vi "Touch_Text.vi"(8 "Error In":errorcluster, 11 "TextTouch":string) -> (0 "error out":errorcluster, 3 "Image":T1(plugin-control))   [LabVIEW 2025]
uses:
  Controls/TextTouch.ctl
  Controls/Text2Img.ctl
  Controls/TouchXY.ctl
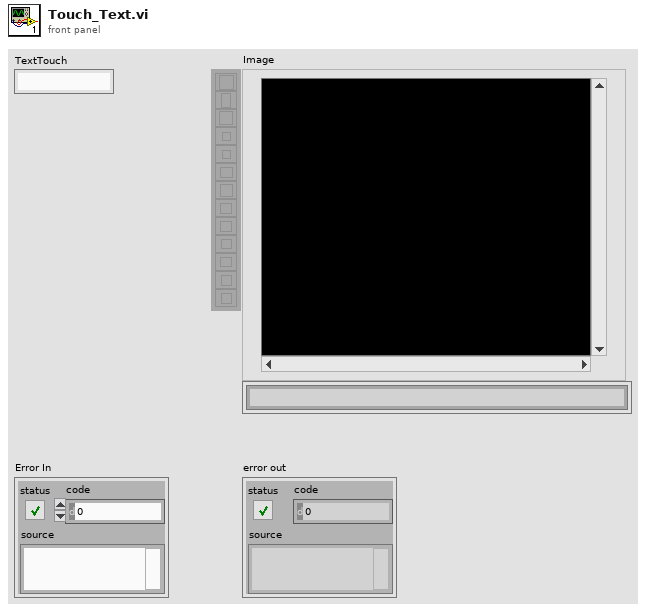
[diagram p1: front panel]
types:
  T1 = typedef "IMAQ Image.ctl" = refnum<image>
  T2 = typedef "TextTouch.ctl" = cluster{"Match%":dbl, "ROI":cluster{"Global Rectangle":i32[], "Contours":cluster{"Contour Type":u32, "ROI Type":u32, "Points":i32[]}[]}, "TextInfo":cluster{"Text":string, "TextColor":cluster{"Text BG":u32, "Text Color":u32}, "Size":u16, "FontDetails":T3}}
  T3 = typedef "Text2Img.ctl" = cluster{"Text.Font":cluster{"Font Name":string, "Size":u16, "Bold":bool, "Italic":bool, "Underline":bool, "Strikeout":bool, "Color":u32}}
  T4 = cluster{"Global Rectangle":i32[], "Contours":cluster{"Contour Type":u32, "ROI Type":u32, "Points":i32[]}[]}
  T5 = cluster{"Text":string, "TextColor":cluster{"Text BG":u32, "Text Color":u32}, "Size":u16, "FontDetails":T3}
  T6 = typedef "TouchXY.ctl" = cluster{"Win Name":string, "TouchCoord":cluster{"x":sgl, "y":sgl}}
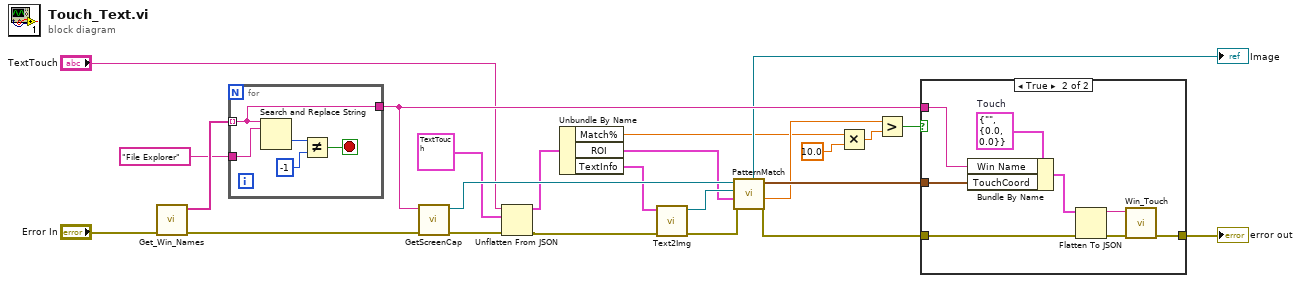
[diagram p0: block diagram]
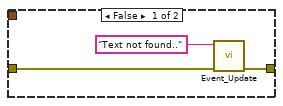
[diagram p2: hidden frame]
diagram:
  n1 = call "Get_Win_Names.vi"("error in"="Error In") -> ("Win_Names"=w23:string[], "error out"=w20:errorcluster)  [unwired: 8 in]
  n2 = for {
    tunnel: w23 -> [w26] mode=indexing
    tunnel: "File Explorer" ("Win Name") -> [w29]
    tunnel: [w26] -> w21
    stop <- w27 stop-if-true
    n3 = Search and Replace String(input string=w26, search string=w29) -> (offset past replacement=w25:i32)  [unwired: 6 in, 3 out]
    n4 = Not Equal?(x=w25, y=-1) -> (x != y?=w27:bool)
  }
  n5 = call "GetScreenCap.vi"("error in (no error)"=w20, "Win Name"=w21) -> ("error out"=w6:errorcluster, "Image Out"=w19:T1)  [unwired: 8 in]
  n6 = Unflatten From JSON(JSON string="TextTouch", type and defaults=T2 {"Match%"=80.0, "ROI"={"Global Rectangle"=[], "Contours"=[]}, "TextInfo"={"Text"="", "TextColor"={"Text BG"=16448250, "Text Color"=0}, "Size"=0, "FontDetails"={"Text.Font"={"Font Name"="Segoe UI", "Size"=29, "Bold"=FALSE, "Italic"=FALSE, "Underline"=FALSE, "Strikeout"=FALSE, "Color"=16448250}}}} ("TextTouch"), error in (no error)=w6) -> (value=w2:T2, error out=w5:errorcluster)  [unwired: 4 in]
  n7 = Unbundle By Name(w2) -> ("Match%"=w11:dbl, "ROI"=w8:T4, "TextInfo"=w1:T5)
  n8 = call "Text2Img.vi"("error in (no error)"=w5, "TextInfo"=w1) -> ("error out"=w7:errorcluster, "Image"=w14:T1)  [unwired: 8 in]
  n9 = call "PatternMatch.vi"("error in"=w7, "ROI"=w8, "Template"=w14, "Image"=w19) -> ("error out"=w18:errorcluster, "Score"=w13:sgl, "Position"=w17:cluster{"x":sgl, "y":sgl}, "Image 2"=→"Image":T1)  [unwired: 3 in, 1 out]
  n10 = Multiply(x=w11, y=10.0) -> (x*y=w9:dbl)
  n11 = Greater?(x=w13, y=w9) -> (0:w12:bool)
  n12 = case shown="True" w12 {
    tunnel: [w31 w40] -> w24
    tunnel: w21 -> [_ w39]
    tunnel: w18 -> [w32 w35]
    tunnel: w17 -> [_ w38]
    frame False {
      n13 = call "Event_Update.vi"("Error In"=w32, "Event"="Text not found..") -> ("Error Out"=w31:errorcluster)  [unwired: 9 in]
    }
    frame True {
      w37 = T6 {"Win Name"="", "TouchCoord"={"x"=0.0, "y"=0.0}}  # Touch
      n14 = Bundle By Name(cluster=w37, "Win Name"=w39, "TouchCoord"=w38) -> (w36:T6)
      n15 = Flatten To JSON(anything=w36, error in (no error)=w35) -> (JSON string=w33:string, 11:w34:errorcluster)  [unwired: 1 in]
      n16 = call "Win_Touch.vi"("error in (no error)"=w34, "TouchXY"=w33) -> ("error out"=w40:errorcluster)  [unwired: 9 in]
    }
  }
  "error out" <- w24
